vi "Validate RaF Custom Device Reference.vi"(8 "error in (no error)":errorcluster, 11 "Routing and Faulting Custom Device Ref in":T1 format="%.0x") -> (0 "error out":errorcluster, 3 "Routing and Faulting Custom Device Ref out":T1 format="%.0x")   [LabVIEW 2017, in "Routing and Faulting Scripting.lvlib"]
uses:
  Routing and Faulting Scripting.lvlib
  <vilib>/NI Veristand/Custom Device API/Custom Device Item Ref.ctl
  Shared/Constants.vi
  Shared/Routing and Faulting Shared.lvlib
  <vilib>/NI VeriStand/Custom Device API/Custom Device API.lvlib
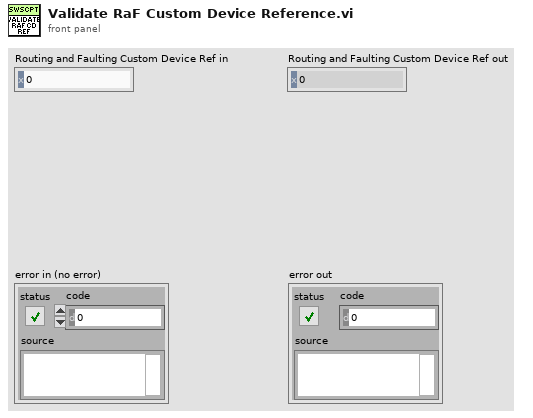
[diagram p1: front panel]
types:
  T1 = typedef "Custom Device API.lvlib/Custom Device Item Ref.ctl" = u64
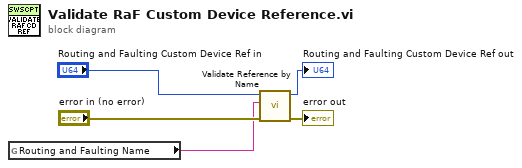
[diagram p0: block diagram]
diagram:
  n1 = global read "Constants.vi" "Routing and Faulting Name"() -> (w1:string)
  n2 = call "Validate Reference by Name.vi"("error in (no error)"="error in (no error)", "Name"=w1, "Ref in"="Routing and Faulting Custom Device Ref in") -> ("error out"=→"error out":errorcluster, "Ref out"=→"Routing and Faulting Custom Device Ref out":T1)  [unwired: 7 in]
